vi "采配水全局变量.vi"() -> ()   [LabVIEW 2016, in "PLC.lvlib"]
uses:
  PLC.lvlib
panel:
  out "空调状态":T1
  out "运行状态显示":string
  out "报警簇":bool[](array[boolean])
  out "参数设置":T2
  in  "状态":T3
  out "转换值":T4
  out "AD":T5
  out "输出状态":bool[](array[boolean])
  out "输入状态":bool[](array[boolean])
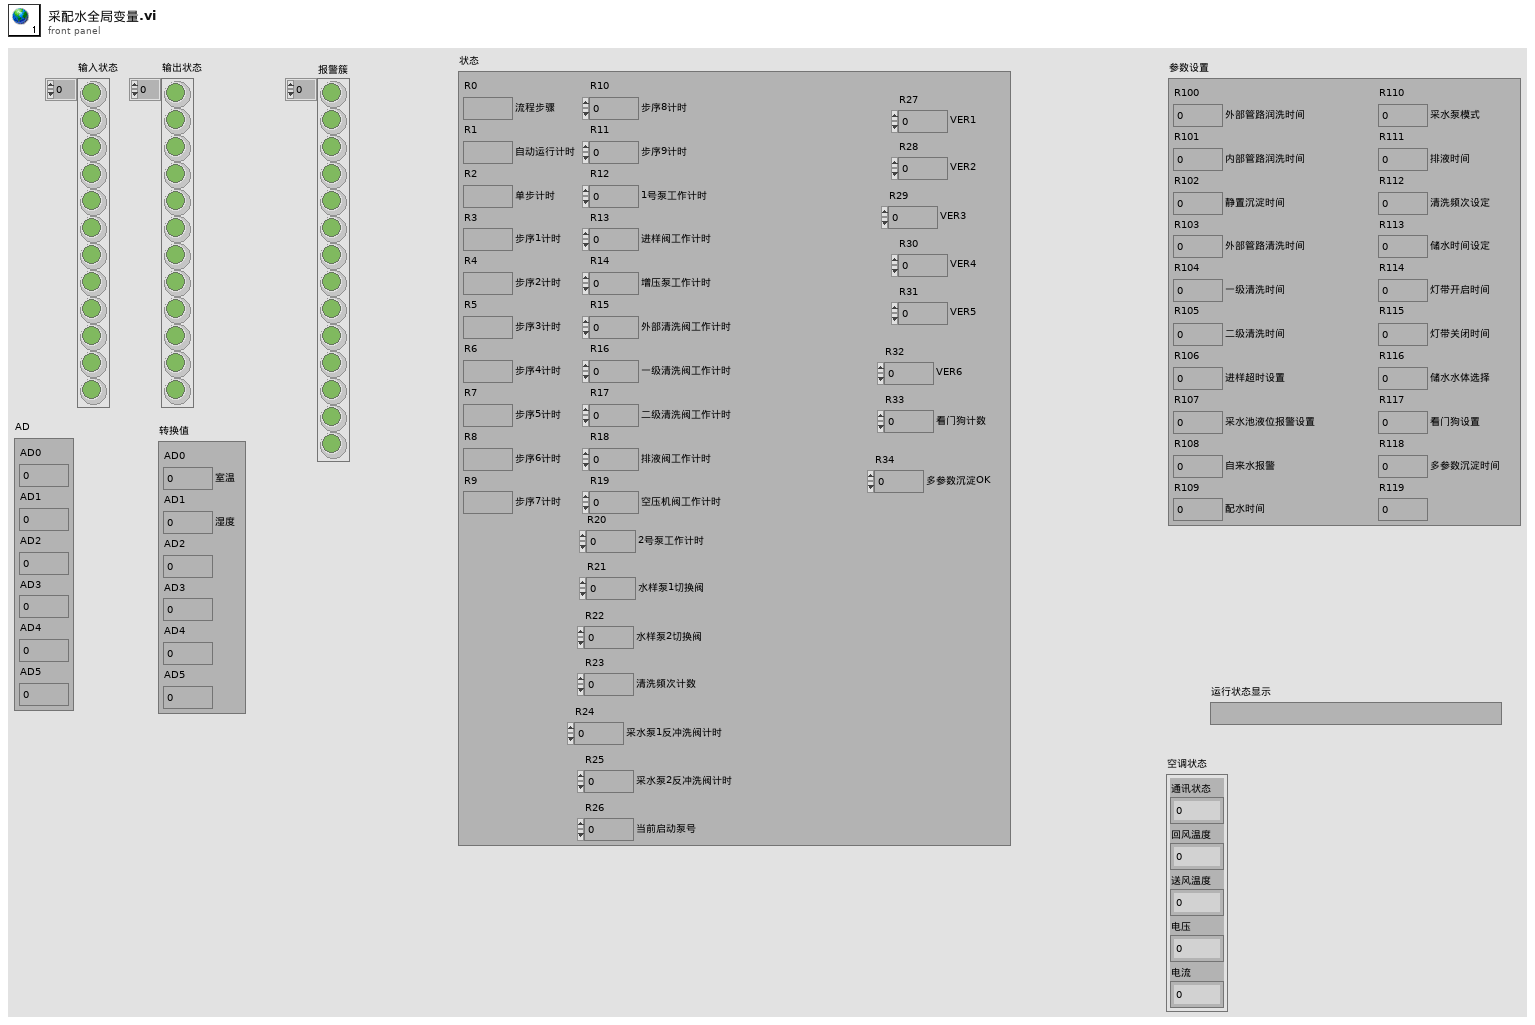
[diagram p1: front panel]
types:
  T1 = cluster{"通讯状态":u16, "回风温度":sgl, "送风温度":sgl, "电压":sgl, "电流":sgl}
  T2 = cluster{"R100":i16, "R101":i16, "R102":i16, "R103":i16, "R104":i16, "R105":i16, "R106":i16, "R107":i16, "R108":i16, "R109":i16, "R110":i16, "R111":i16, "R112":i16, "R113":i16, "R114":i16, "R115":i16, "R116":i16, "R117":i16, "R118":i16, "R119":i16}
  T3 = cluster{"R0":i16, "R1":i16, "R2":i16, "R3":i16, "R4":i16, "R5":i16, "R6":i16, "R7":i16, "R8":i16, "R9":i16, "R10":i16, "R11":i16, "R12":i16, "R13":i16, "R14":i16, "R15":i16, "R16":i16, "R17":i16, "R18":i16, "R19":i16, "R20":i16, "R21":i16, "R22":i16, "R23":i16, "R24":i16, "R25":i16, "R26":i16, "R27":i16, "R28":i16, "R29":i16, "R30":i16, "R31":i16, "R32":i16, "R33":i16, "R34":i16}
  T4 = cluster{"AD0":sgl, "AD1":sgl, "AD2":sgl, "AD3":sgl, "AD4":sgl, "AD5":sgl}
  T5 = cluster{"AD0":i16, "AD1":i16, "AD2":i16, "AD3":i16, "AD4":i16, "AD5":i16}
diagram:
